vi "InterfaceNode_GetAttributesToModify.vi"(0 "reference in":refnum<class "InterfaceNode.lvclass">, 3 "timeout (15000 ms)":i32=15000, 5 "error in (no error)":errorcluster) -> (14 "reference out":refnum<class "InterfaceNode.lvclass">, 16 "Attributes":T1 {"botHeight" format="%.2f"; "midHeight" format="%.2f"; "Base class"."bounds"."height" format="%.2f"; "Base class"."bounds"."width" format="%.2f"; "Base class"."bounds"."y" format="%.2f"; "Base class"."bounds"."x" format="%.2f"}, 17 "Timeout":bool, 19 "error out":errorcluster)   [LabVIEW 2014, in "InterfaceNode.lvclass"]
doc: "This VI returns the attributes associated with the InterfaceNode object reference and places a lock on the object.\n\nIf the object is currently locked for modification by another method, 'Timeout' specifies how long the VI should wait to receive access to the object. The default value waits until the object becomes available.\n\nYou must use the InterfaceNode SetModifiedAttributes VI to set the object's data and release the lock.\n\n[GOOP 2.0.15]"
uses:
  <resource>/Framework/Providers/Open_GDS/UML/InterfaceNode_class/InterfaceNode.lvclass
  <resource>/Framework/Providers/Open_GDS/UML/InterfaceNode_class/protected/ObjectAttributes.ctl
  <resource>/Framework/Providers/Open_GDS/UML/AbstractNode_class/AbstractNode.lvclass
  <resource>/Framework/Providers/Open_GDS/UML/MultiLineString_class/MultiLineString.lvclass
  <resource>/Framework/Providers/Open_GDS/UML/RectangularNode_class/protected/ObjectAttributes.ctl
  <resource>/Framework/Providers/Open_GDS/UML/AbstractNode_class/protected/ObjectAttributes.ctl
  <resource>/Framework/Providers/Open_GDS/UML/General/Rectangle/Rectangle Rectangle2D.ctl
  <vilib>/addons/_goop3.llb/3GOOPStates.ctl
  <resource>/Framework/Providers/Open_GDS/UML/InterfaceNode_class/InterfaceNode.lvclass/InterfaceNode.ctl
  <resource>/Framework/Providers/Open_GDS/UML/RectangularNode_class/RectangularNode.lvclass
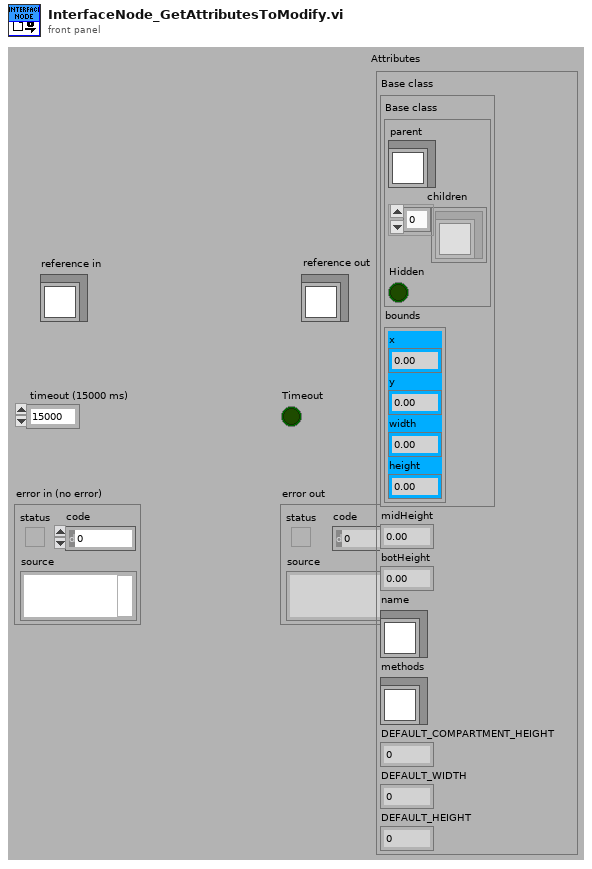
[diagram p1: front panel]
types:
  T1 = typedef "InterfaceNode.lvclass/ObjectAttributes.ctl" = cluster{"Base class":T2, "midHeight":dbl, "botHeight":dbl, "name":refnum<class "MultiLineString.lvclass">, "methods":refnum<class "MultiLineString.lvclass">, "DEFAULT_COMPARTMENT_HEIGHT":i32, "DEFAULT_WIDTH":i32, "DEFAULT_HEIGHT":i32}
  T2 = typedef "RectangularNode.lvclass/ObjectAttributes.ctl" = cluster{"Base class":T3, "bounds":T4}
  T3 = typedef "AbstractNode.lvclass/ObjectAttributes.ctl" = cluster{"parent":refnum<class "AbstractNode.lvclass">, "children":refnum<class "AbstractNode.lvclass">[], "Hidden":bool}
  T4 = typedef "Rectangle Rectangle2D.ctl" = cluster{"x":dbl, "y":dbl, "width":dbl, "height":dbl}
  T5 = typedef "3GOOPStates.ctl" = enum16{"Set", "Get", "New", "Delete", "Clear", "Test and get", "Unlock data", "Information", "Look up existing", "New or look up existing", "Test and get shared", "Get shared", "Set shared", "Unlock shared", "Find dynamic method", "Register dynamic method", "Preload dynamic method", "Probe", "Cast to more generic", "Cast to more specific"}
  T6 = typedef "AbstractNode.lvclass/ObjectReference.ctl" = refnum<k1>
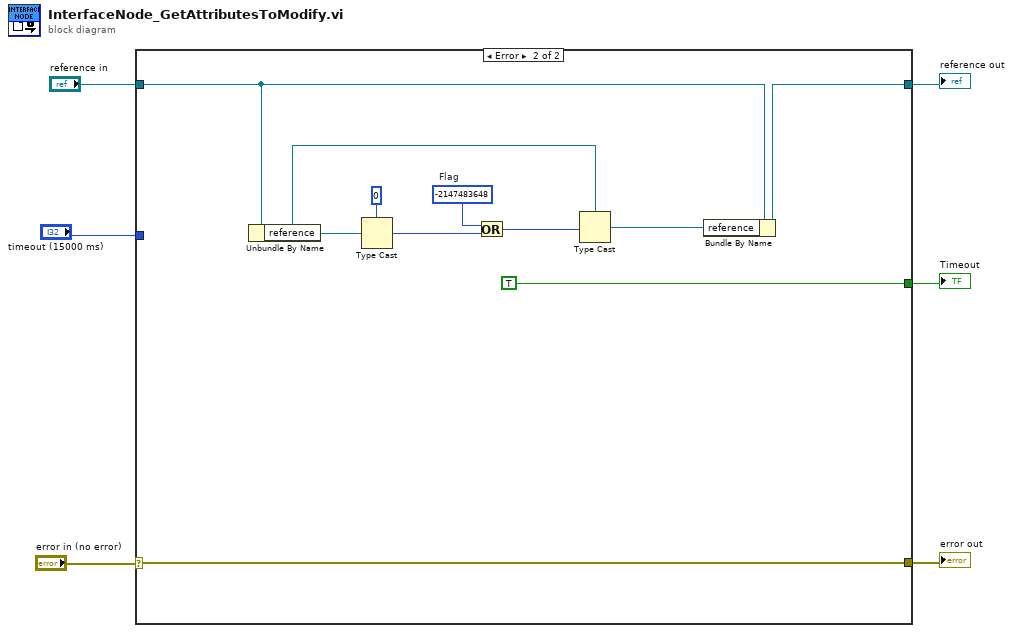
[diagram p0: block diagram]
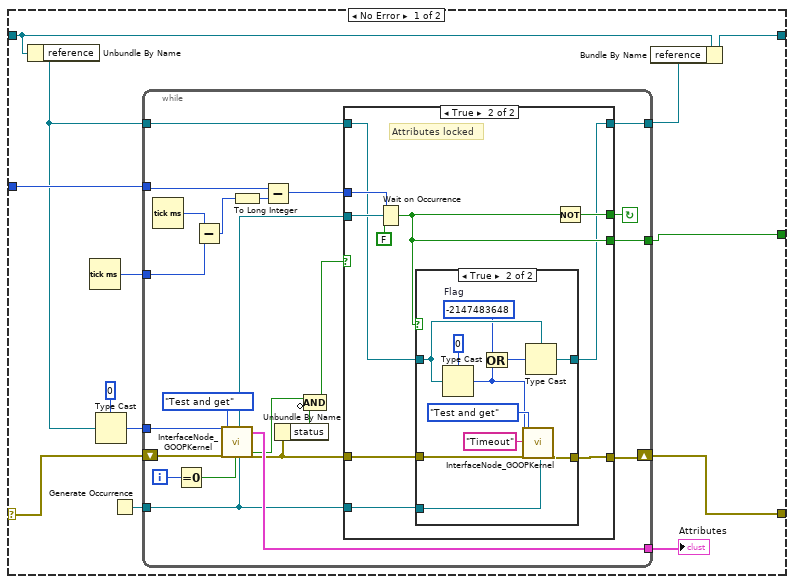
[diagram p2: hidden frame]
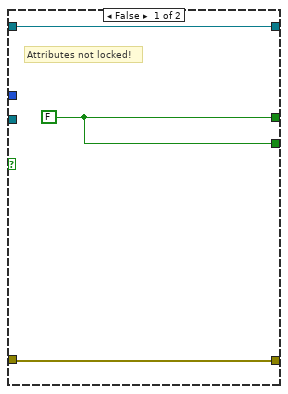
[diagram p3: hidden frame]
diagram:
  n1 = case shown="Error" "error in (no error)" {
    selector: "error in (no error)" -> [w14 w78]
    tunnel: [w9 w69] -> w3
    tunnel: [w13 w78] -> w1
    tunnel: "reference in" -> [w10 w70]
    tunnel: [w12 TRUE ("timed out")] -> w2
    tunnel: "timeout (15000 ms)" -> [w15 _]
    frame No Error {
      n2 = Unbundle By Name(w10) -> ("reference"=w11:T6)
      n3 = Tick Count (ms)() -> (millisecond timer value=w16:u32)
      n4 = Type Cast(type=0, x=w11) -> (*(type *) &x=w19:i32)
      n5 = Generate Occurrence() -> (w17:refnum<k4>)
      n6 = while {
        tunnel: [w38] -> w7
        shift-left: w14 -> [w39]
        shift-right: [w24] -> w13
        tunnel: [w41] -> w12
        tunnel: w15 -> [w30]
        tunnel: w19 -> [w40]
        tunnel: w17 -> [w23]
        tunnel: w16 -> [w20]
        tunnel: w11 -> [w26]
        tunnel: [w22] -> w8
        i -> [w34]
        stop <- w42 continue-if-true
        n7 = Tick Count (ms)() -> (millisecond timer value=w21:u32)
        n8 = Equal To 0?(x=w34) -> (x = 0?=w33:bool)
        n9 = Subtract(x=w21, y=w20) -> (x-y=w29:u32)
        n10 = call <resource>:"InterfaceNode_GOOPKernel.vi"("Ref in"=w40, "error in (no error)"=w39, "Action"=3GOOPStates."Test and get", "First try?"=w33, "Occurrence"=w23) -> ("Occurrence out"=w32:refnum<k4>, "Data out"=w38:T1, "Data locked?"=w36:bool, "error out"=w25:errorcluster)  [unwired: 10 in, 9 out]
        n11 = To Long Integer(number=w29) -> (32bit integer=w27:i32)
        n12 = Subtract(x=w30, y=w27) -> (x-y=w28:i32)
        n13 = Unbundle By Name(w25) -> ("status"=w37:bool)
        n14 = Compound Arithmetic op=AND(w36, invert w37) -> (w35:bool)
        n15 = case shown="True" w35 {
          tunnel: w32 -> [_ w54]
          tunnel: w28 -> [_ w52]
          tunnel: [w45 w55] -> w42
          tunnel: [w45 w48] -> w41
          tunnel: w26 -> [w43 w51]
          tunnel: w25 -> [w44 w50]
          tunnel: [w44 w49] -> w24
          tunnel: w23 -> [_ w47]
          tunnel: [w43 w46] -> w22
          frame False {
            w45 = FALSE
            # "Attributes not locked!"
          }
          frame True {
            # "Attributes locked"
            n16 = Wait on Occurrence(1:FALSE ("ignore previous (T)"), 2:w54, 3:w52) -> (0:w48:bool)
            n17 = case shown="True" w48 {
              tunnel: w51 -> [w56 w61]
              tunnel: w50 -> [w57 w68]
              tunnel: [w57 w67] -> w49
              tunnel: w47 -> [_ w64]
              tunnel: [w56 w60] -> w46
              frame False {
              }
              frame True {
                w58 = -2147483648  # Flag
                n18 = Type Cast(type=0, x=w61) -> (*(type *) &x=w62:i32)
                n19 = Or(x=w58, y=w62) -> (x .or. y?=w63:i32)
                n20 = call <resource>:"InterfaceNode_GOOPKernel.vi"("Ref in"=w62, "VI ref"="Timeout", "error in (no error)"=w68, "Action"=3GOOPStates."Test and get", "Occurrence"=w64) -> ("error out"=w67:errorcluster)  [unwired: 10 in, 12 out]
                n21 = Type Cast(type=w61, x=w63) -> (*(type *) &x=w60:T6)
              }
            }
            n22 = Not(x=w48) -> (.not. x?=w55:bool)
          }
        }
      }
      "Attributes" <- w7
      n23 = Bundle By Name(cluster=w10, "reference"=w8) -> (w9:refnum<class "InterfaceNode.lvclass">)
    }
    frame Error {
      w74 = -2147483648  # Flag
      n24 = Unbundle By Name(w70) -> ("reference"=w72:T6)
      n25 = Type Cast(type=0, x=w72) -> (*(type *) &x=w75:i32)
      n26 = Or(x=w74, y=w75) -> (x .or. y?=w73:i32)
      n27 = Type Cast(type=w72, x=w73) -> (*(type *) &x=w71:T6)
      n28 = Bundle By Name(cluster=w70, "reference"=w71) -> (w69:refnum<class "InterfaceNode.lvclass">)
    }
  }
  "error out" <- w1
  "reference out" <- w3
  "Timeout" <- w2
